vi "calibration.vi"(11 "输入簇":T2) -> ()   [LabVIEW 2018]
uses:
  global.vi
panel:
  in  "正在校准":string
  in  "开始校准":T1
  out "MIC4":waveform(dbl)(graph)
  out "MIC3":waveform(dbl)(graph)
  out "MIC1":waveform(dbl)(graph)
  out "MIC2":waveform(dbl)(graph)
  # "step1：将传声器插入校准器，\n             点击\"开始校准\"按钮"
  # "step2：将麦克风按照图中位置放置"
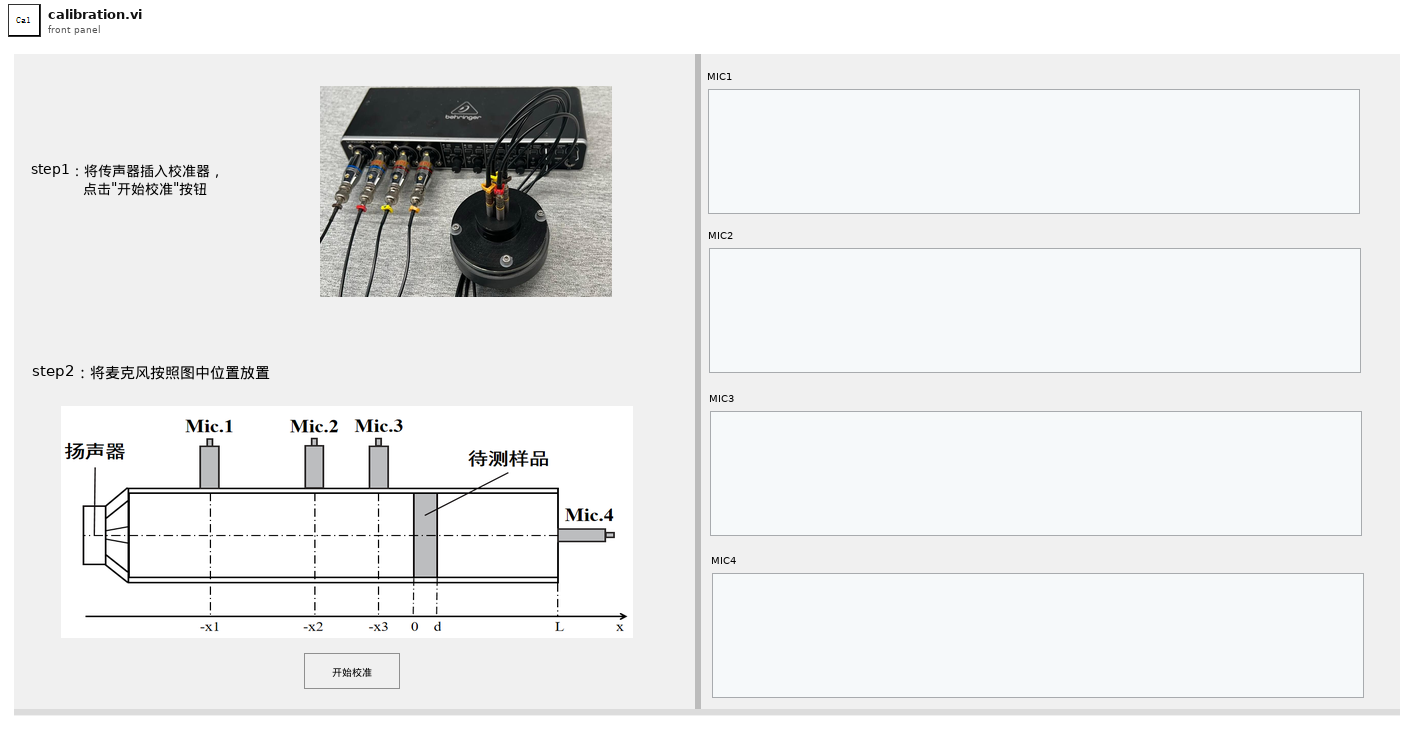
[diagram p1: front panel]
types:
  T1 = typedef "布尔控件.ctl" = bool
  T2 = cluster{"幅值(V)":dbl, "信号时长(s)":dbl, "频率上限(Hz)":dbl, "频率下限(Hz)":dbl}
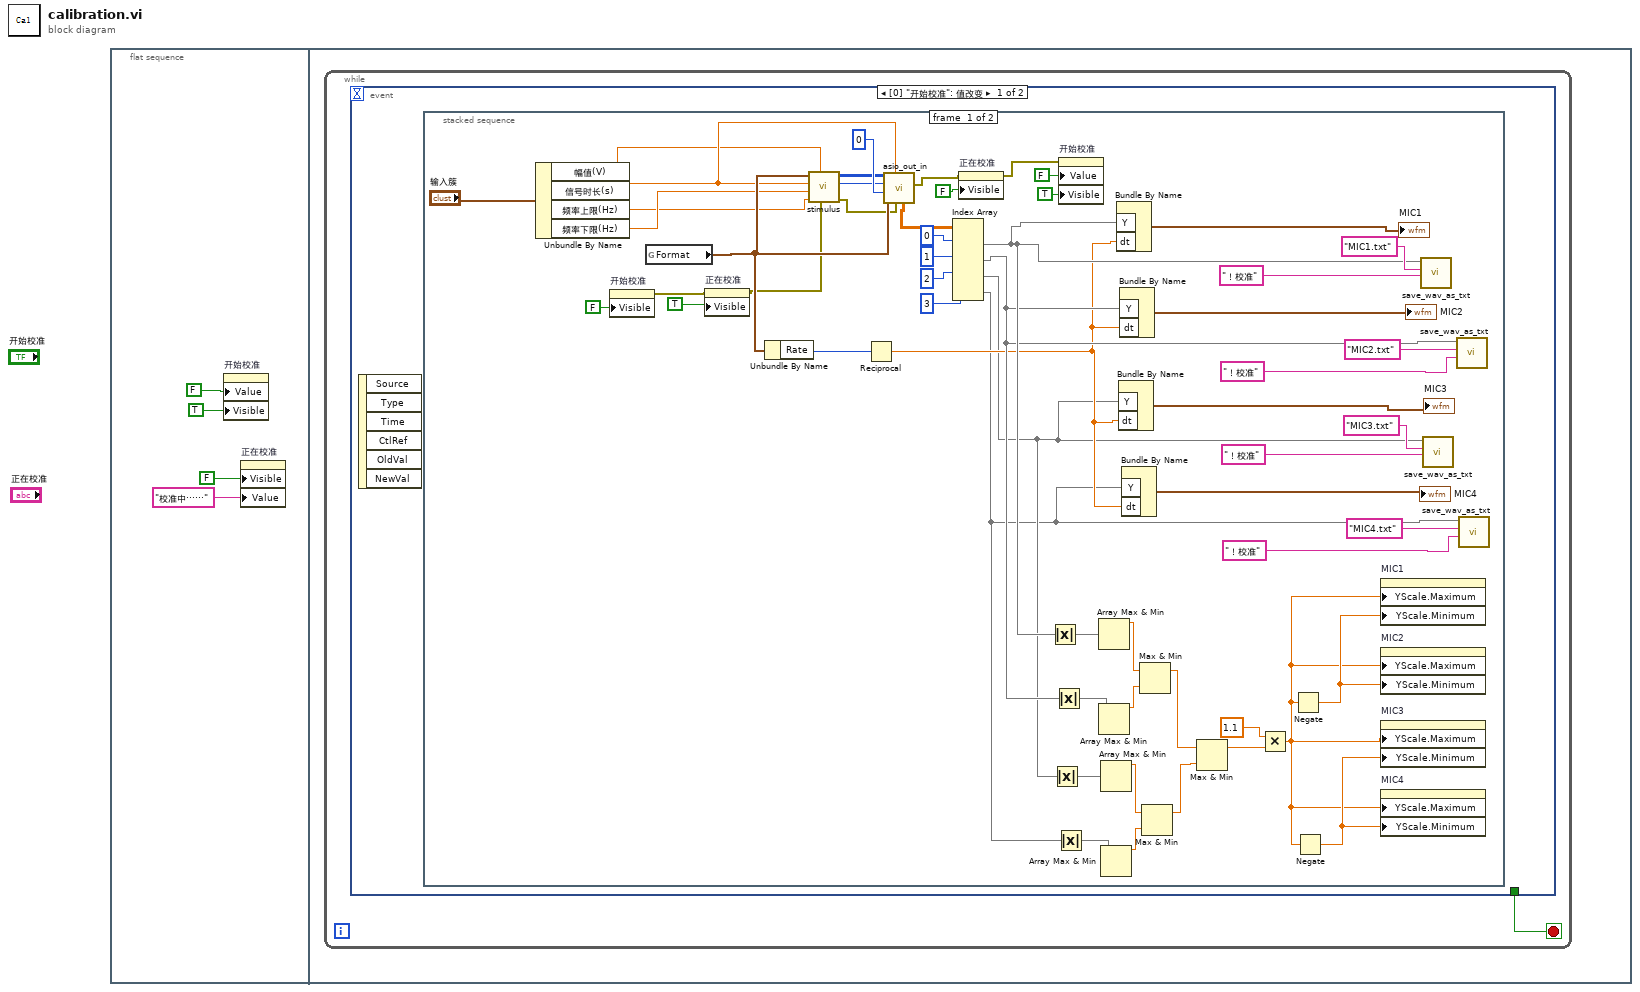
[diagram p0: block diagram]
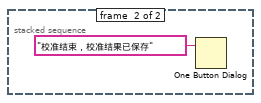
[diagram p2: hidden frame]
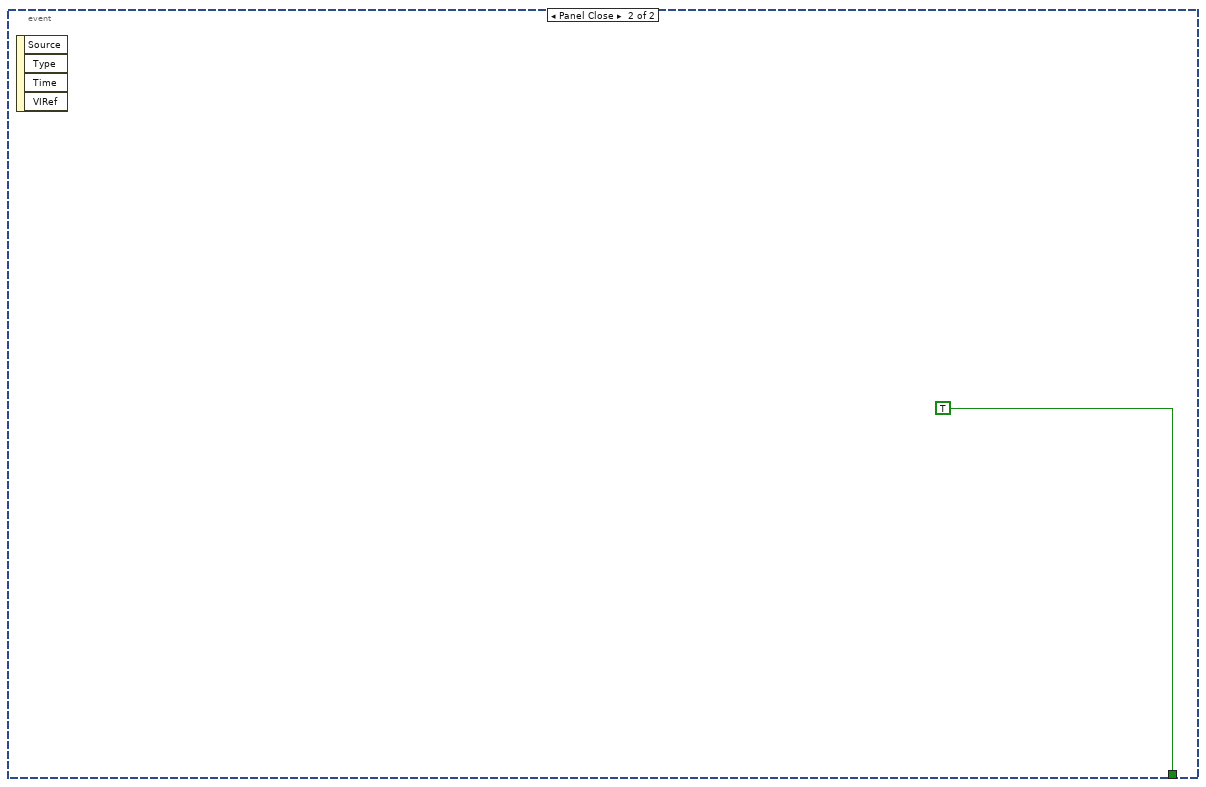
[diagram p3: hidden frame]
diagram:
  n1 = flat-sequence {
    frame #0 {
      n2 = property on="开始校准" class="Bool (严格)"("Value"=T1 FALSE ("开始校准"), "Visible"=TRUE ("可见")) -> ()  [unwired: 2 in, 2 out]
      n3 = property on="正在校准" class="Str"("Visible"=FALSE ("可见"), "Value"="校准中······" ("校准中")) -> ()  [unwired: 2 in, 2 out]
    }
    frame #1 {
      n4 = while {
        stop <- w5 stop-if-true
        n5 = event shown="[0] \"开始校准\": 值改变" {
          selector: _ -> [_ _]
          dyn-events: _ -> [_ _]
          timeout: _ -> [_ _]
          tunnel: [_ TRUE] -> w5
          event Value Change {
            n6 = event-data() -> ()  [unwired: 1 in, 6 out]
            n7 = stacked-sequence {
              frame #0 {
                n8 = Unbundle By Name("输入簇") -> ("幅值(V)"=w50:dbl, "信号时长(s)"=w53:dbl, "频率上限(Hz)"=w51:dbl, "频率下限(Hz)"=w52:dbl)
                n9 = property on="开始校准" class="Bool (严格)"("Visible"=FALSE ("可见")) -> (error out=w36:errorcluster)  [unwired: 2 in, 1 out]
                n10 = global read "global.vi" "Format"() -> (w57:cluster{"Rate":i32, "Bits":i32, "Channels":u32})
                n11 = property on="正在校准" class="Str"(error in=w36, "Visible"=TRUE ("可见")) -> (error out=w35:errorcluster)  [unwired: 1 in, 1 out]
                n12 = Unbundle By Name(w57) -> ("Rate"=w58:i32)
                n13 = call "stimulus.vi"("error play 2"=w35, "幅值(V)"=w50, "stop frequency [Hz]"=w51, "start frequency [Hz]"=w52, "信号时长"=w53, "Format"=w57) -> ("error play 3"=w44:errorcluster, "data length"=w48:i32, "Output data"=w47:i32[][])  [unwired: 2 in, 1 out]
                n14 = Reciprocal(x=w58) -> (1/x=w14:dbl)
                n15 = call "asio_out_in.vi"("error play 4"=w44, "信号时长"=w53, "Format"=w57, "card #"=u32 0, "data_length"=w48, "output data"=w47) -> ("error play 2"=w39:errorcluster, "MIC_Data_IN"=w54:dbl[][])  [unwired: 3 in, 1 out]
                n16 = Index Array(array=w54, index (row) #1=0 ("索引 (行)"), index (row) #2=1 ("索引 (行)"), index (row) #3=2 ("索引 (行)"), index (row) #4=3 ("索引 (行)")) -> (element #1=w30:dbl[], element #2=w28:dbl[], element #3=w11:dbl[], element #4=w10:dbl[])  [unwired: 4 in]
                n17 = property on="正在校准" class="Str"(error in=w39, "Visible"=FALSE ("可见")) -> (error out=w38:errorcluster)  [unwired: 1 in, 1 out]
                n18 = Absolute Value(x=w30) -> (abs(x)=w29:dbl[])
                n19 = Absolute Value(x=w11) -> (abs(x)=w19:dbl[])
                n20 = Absolute Value(x=w28) -> (abs(x)=w27:dbl[])
                n21 = Absolute Value(x=w10) -> (abs(x)=w20:dbl[])
                n22 = property on="开始校准" class="Bool (严格)"(error in=w38, "Value"=T1 FALSE ("开始校准"), "Visible"=T1 TRUE ("开始校准")) -> ()  [unwired: 1 in, 2 out]
                n23 = Array Max & Min(array=w29) -> (max value=w31:dbl)  [unwired: 3 out]
                n24 = Array Max & Min(array=w27) -> (max value=w32:dbl)  [unwired: 3 out]
                n25 = Array Max & Min(array=w19) -> (max value=w18:dbl)  [unwired: 3 out]
                n26 = Array Max & Min(array=w20) -> (max value=w17:dbl)  [unwired: 3 out]
                n27 = Bundle By Name("Y"=w30, "dt"=w14) -> (→"MIC1":waveform(dbl))  [unwired: 1 in]
                n28 = Bundle By Name("Y"=w11, "dt"=w14) -> (→"MIC3":waveform(dbl))  [unwired: 1 in]
                n29 = Bundle By Name("Y"=w28, "dt"=w14) -> (→"MIC2":waveform(dbl))  [unwired: 1 in]
                n30 = Bundle By Name("Y"=w10, "dt"=w14) -> (→"MIC4":waveform(dbl))  [unwired: 1 in]
                n31 = Max & Min(x=w31, y=w32) -> (max(x,y)=w9:dbl)  [unwired: 1 out]
                n32 = Max & Min(x=w18, y=w17) -> (max(x,y)=w8:dbl)  [unwired: 1 out]
                n33 = Max & Min(x=w9, y=w8) -> (max(x,y)=w7:dbl)  [unwired: 1 out]
                n34 = Multiply(x=1.1, y=w7) -> (x*y=w6:dbl)
                n35 = Negate(x=w6) -> (-x=w26:dbl)
                n36 = Negate(x=w6) -> (-x=w21:dbl)
                n37 = property on="MIC1" class="WFGraph (严格)"("YScale.Maximum"=w6, "YScale.Minimum"=w26) -> ()  [unwired: 2 in, 2 out]
                n38 = property on="MIC2" class="WFGraph (严格)"("YScale.Maximum"=w6, "YScale.Minimum"=w26) -> ()  [unwired: 2 in, 2 out]
                n39 = property on="MIC3" class="WFGraph (严格)"("YScale.Maximum"=w6, "YScale.Minimum"=w21) -> ()  [unwired: 2 in, 2 out]
                n40 = property on="MIC4" class="WFGraph (严格)"("YScale.Maximum"=w6, "YScale.Minimum"=w21) -> ()  [unwired: 2 in, 2 out]
                n41 = call "save_wav_as_txt.vi"("文件夹名"="！校准", "txt名"="MIC1.txt", "wav"=w30) -> ()  [unwired: 9 in]
                n42 = call "save_wav_as_txt.vi"("文件夹名"="！校准", "txt名"="MIC3.txt", "wav"=w11) -> ()  [unwired: 9 in]
                n43 = call "save_wav_as_txt.vi"("文件夹名"="！校准", "txt名"="MIC2.txt", "wav"=w28) -> ()  [unwired: 9 in]
                n44 = call "save_wav_as_txt.vi"("文件夹名"="！校准", "txt名"="MIC4.txt", "wav"=w10) -> ()  [unwired: 9 in]
              }
              frame #1 {
                n45 = One Button Dialog(message="校准结束，校准结果已保存" ("消息")) -> ()  [unwired: 1 in, 1 out]
              }
            }
          }
          event Panel Close {
            n46 = event-data() -> ()  [unwired: 1 in, 4 out]
          }
        }
      }
    }
  }
